vi "FB Switch Output No Term Var Write.vi"(8 "error in":errorcluster, 11 "data in":variant) -> (0 "error out":errorcluster)   [LabVIEW 2020]
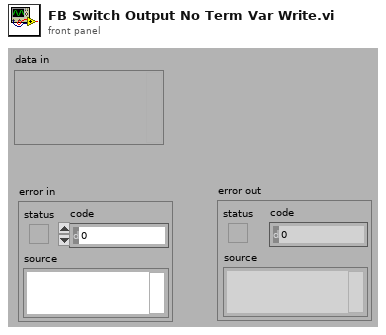
[diagram p1: front panel]
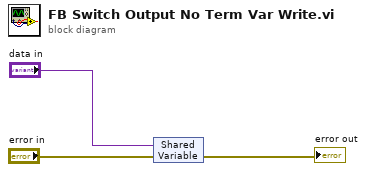
[diagram p0: block diagram]
diagram:
  n1 = shared-variable("data in", error in="error in") -> (error out=→"error out":errorcluster)
